vi "SoundRocket.vi"   [LabVIEW 2013]
types:
  T1 = typedef "Sound Output Task ID.ctl" = u32
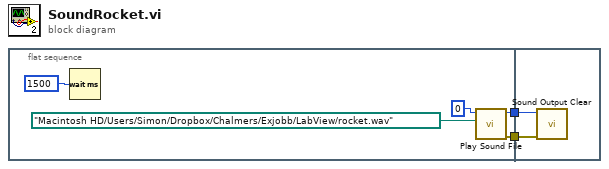
[diagram p0: block diagram]
diagram:
  n1 = flat-sequence {
    tunnel: [w6] -> w2
    tunnel: [w5] -> w1
    tunnel: w2 -> [w9]
    tunnel: w1 -> [w8]
    frame #0 {
      n2 = Wait (ms)(milliseconds to wait=u32 1500) -> ()  [unwired: 1 out]
      n3 = call <vilib>:"Play Sound File.vi"("path"=path "/Macintosh HD/Users/Simon/Dropbox/Chalmers/Exjobb/LabView/rocket.wav", "device ID"=u32 0) -> ("error out"=w6:errorcluster, "task ID"=w5:T1)  [unwired: 8 in]
    }
    frame #1 {
      n4 = call <vilib>:"Sound Output Clear.vi"("error in (no error)"=w9, "task ID"=w8) -> ()  [unwired: 9 in, 1 out]
    }
  }
